vi "JSONtext Multi-step Filter.vi"() -> ()   [LabVIEW 2017] (continued)
: \"2014-12-13T11:18:37 -00:00\",\n    \"latitude\": 44.611706,\n    \"longitude\": -75.982853,\n    \"tags\": [\n      \"non\",\n      \"mollit\",\n      \"pariatur\",\n      \"ad\",\n      \"aliqua\",\n      \"do\",\n      \"laboris\"\n    ],\n    \"friends\": [\n      {\n        \"id\": 0,\n        \"name\": \"Cannon Navarro\"\n      },\n      {\n        \"id\": 1,\n        \"name\": \"Terri Byers\"\n      },\n      {\n        \"id\": 2,\n        \"name\": \"Janell Robinson\"\n      }\n    ],\n    \"greeting\": \"Hello, Carroll Kline! You have 4 unread messages.\",\n    \"favoriteFruit\": \"banana\"\n  },\n  {\n    \"_id\": \"59b53bcb034cefc38e5f718d\",\n    \"index\": 14,\n    \"guid\": \"1b75941b-966f-4520-bda0-746f5f72a03e\",\n    \"isActive\": false,\n    \"balance\": \"$2,799.30\",\n    \"picture\": \"http://placehold.it/32x32\",\n    \"age\": 32,\n    \"eyeColor\": \"brown\",\n    \"name\": \"Forbes Tran\",\n    \"gender\": \"male\",\n    \"company\": \"LYRIA\",\n    \"email\": \"forbestran@lyria.com\",\n    \"phone\": \"+1 (932) 582-3482\",\n    \"address\": \"689 Cook Street, Cleary, Iowa, 2553\",\n    \"about\": \"Occaecat tempor sint nisi amet ex veniam culpa adipisicing ad. Incididunt duis elit amet deserunt eiusmod officia occaecat eiusmod qui incididunt. Eiusmod laboris esse sit incididunt enim eu excepteur est mollit anim ad quis. Mollit nulla culpa veniam incididunt ipsum sit officia sunt aliqua reprehenderit dolor dolore. Culpa excepteur consequat magna elit id ullamco deserunt est in et irure.\\r\\n\",\n    \"registered\": \"2015-05-22T09:52:23 -01:00\",\n    \"latitude\": 9.60954,\n    \"longitude\": -42.310375,\n    \"tags\": [\n      \"mollit\",\n      \"proident\",\n      \"veniam\",\n      \"irure\",\n      \"esse\",\n      \"Lorem\",\n      \"dolore\"\n    ],\n    \"friends\": [\n      {\n        \"id\": 0,\n        \"name\": \"Leila Sims\"\n      },\n      {\n        \"id\": 1,\n        \"name\": \"Desiree Savage\"\n      },\n      {\n        \"id\": 2,\n        \"name\": \"Johnston Hensley\"\n      }\n    ],\n    \"greeting\": \"Hello, Forbes Tran! You have 3 unread messages.\",\n    \"favoriteFruit\": \"banana\"\n  },\n  {\n    \"_id\": \"59b53bcb9a6e9676f507278e\",\n    \"index\": 15,\n    \"guid\": \"3bed5db5-ef23-4804-a3e0-08b3c940d53f\",\n    \"isActive\": true,\n    \"balance\": \"$1,219.22\",\n    \"picture\": \"http://placehold.it/32x32\",\n    \"age\": 39,\n    \"eyeColor\": \"brown\",\n    \"name\": \"Carlson Klein\",\n    \"gender\": \"male\",\n    \"company\": \"AQUACINE\",\n    \"email\": \"carlsonklein@aquacine.com\",\n    \"phone\": \"+1 (978) 572-2330\",\n    \"address\": \"863 Woods Place, Movico, Wyoming, 810\",\n    \"about\": \"Do excepteur nostrud est nisi minim incididunt cillum. Et veniam do in proident deserunt minim sit. Sunt pariatur ipsum tempor elit duis sint sit non non qui laborum duis esse. Sint eiusmod irure pariatur occaecat reprehenderit anim.\\r\\n\",\n    \"registered\": \"2014-05-03T11:19:28 -01:00\",\n    \"latitude\": -56.803333,\n    \"longitude\": -128.863204,\n    \"tags\": [\n      \"tempor\",\n      \"velit\",\n      \"voluptate\",\n      \"et\",\n      \"laboris\",\n      \"consequat\",\n      \"cillum\"\n    ],\n    \"friends\": [\n      {\n        \"id\": 0,\n        \"name\": \"Liliana Sellers\"\n      },\n      {\n        \"id\": 1,\n        \"name\": \"Garcia Larsen\"\n      },\n      {\n        \"id\": 2,\n        \"name\": \"Long Fitzpatrick\"\n      }\n    ],\n    \"greeting\": \"Hello, Carlson Klein! You have 4 unread messages.\",\n    \"favoriteFruit\": \"strawberry\"\n  },\n  {\n    \"_id\": \"59b53bcbac141192de4ff36f\",\n    \"index\": 16,\n    \"guid\": \"5c96733c-76df-40fa-b2b3-d65d58dc0720\",\n    \"isActive\": true,\n    \"balance\": \"$2,144.12\",\n    \"picture\": \"http://placehold.it/32x32\",\n    \"age\": 38,\n    \"eyeColor\": \"blue\",\n    \"name\": \"Maryann Adams\",\n    \"gender\": \"female\",\n    \"company\": \"GEEKY\",\n    \"email\": \"maryannadams@geeky.com\",\n    \"phone\": \"+1 (814) 507-3036\",\n    \"address\": \"701 Albemarle Terrace, Datil, Marshall Islands, 1322\",\n    \"about\": \"Ipsum velit nostrud minim aute velit ut esse occaecat ad voluptate qui ad. Mollit pariatur ullamco Lorem quis elit incididunt anim ullamco officia laborum. Ad incididunt ut ipsum elit elit culpa magna. Nulla quis ex est elit commodo deserunt culpa culpa sint occaecat do. Consectetur irure officia culpa id ex. Et est id minim proident Lorem ea esse aute et qui. Quis enim duis minim sint elit nostrud.\\r\\n\",\n    \"registered\": \"2016-11-20T04:37:14 -00:00\",\n    \"latitude\": -61.054651,\n    \"longitude\": -110.864468,\n    \"tags\": [\n      \"excepteur\",\n      \"minim\",\n      \"amet\",\n      \"magna\",\n      \"fugiat\",\n      \"excepteur\",\n      \"consectetur\"\n    ],\n    \"friends\": [\n      {\n        \"id\": 0,\n        \"name\": \"Megan Petersen\"\n      },\n      {\n        \"id\": 1,\n        \"name\": \"Arline Solis\"\n      },\n      {\n        \"id\": 2,\n        \"name\": \"Carpenter Bishop\"\n      }\n    ],\n    \"greeting\": \"Hello, Maryann Adams! You have 4 unread messages.\",\n    \"favoriteFruit\": \"apple\"\n  },\n  {\n    \"_id\": \"59b53bcbd4794b54dacb02ff\",\n    \"index\": 17,\n    \"guid\": \"9b12691d-534a-49ef-9453-e6db5e086fa3\",\n    \"isActive\": true,\n    \"balance\": \"$1,444.83\",\n    \"picture\": \"http://placehold.it/32x32\",\n    \"age\": 23,\n    \"eyeColor\": \"brown\",\n    \"name\": \"Zelma Hooper\",\n    \"gender\": \"female\",\n    \"company\": \"ENDICIL\",\n    \"email\": \"zelmahooper@endicil.com\",\n    \"phone\": \"+1 (953) 529-2225\",\n    \"address\": \"327 Cherry Street, Sylvanite, Nevada, 1609\",\n    \"about\": \"Aliquip consectetur dolor magna irure voluptate ea. Labore id aute incididunt eiusmod ad cillum est exercitation excepteur officia cupidatat aute. Sit et magna duis duis excepteur ad est sit sint adipisicing commodo. Sint est quis amet ullamco cupidatat nisi enim sint do et.\\r\\n\",\n    \"registered\": \"2015-10-10T05:49:22 -01:00\",\n    \"latitude\": -69.361083,\n    \"longitude\": -9.671064,\n    \"tags\": [\n      \"veniam\",\n      \"officia\",\n      \"dolore\",\n      \"dolore\",\n      \"occaecat\",\n      \"excepteur\",\n      \"dolore\"\n    ],\n    \"friends\": [\n      {\n        \"id\": 0,\n        \"name\": \"Hughes Mcgowan\"\n      },\n      {\n        \"id\": 1,\n        \"name\": \"Corrine Velazquez\"\n      },\n      {\n        \"id\": 2,\n        \"name\": \"Wade Kirkland\"\n      }\n    ],\n    \"greeting\": \"Hello, Zelma Hooper! You have 6 unread messages.\",\n    \"favoriteFruit\": \"strawberry\"\n  },\n  {\n    \"_id\": \"59b53bcb68e219d872f06a49\",\n    \"index\": 18,\n    \"guid\": \"861c801f-0f15-4390-8104-311e6d6f83d8\",\n    \"isActive\": true,\n    \"balance\": \"$2,222.35\",\n    \"picture\": \"http://placehold.it/32x32\",\n    \"age\": 34,\n    \"eyeColor\": \"green\",\n    \"name\": \"Gwen Cook\",\n    \"gender\": \"female\",\n    \"company\": \"BESTO\",\n    \"email\": \"gwencook@besto.com\",\n    \"phone\": \"+1 (999) 515-3826\",\n    \"address\": \"151 Wythe Place, Hessville, North Carolina, 3410\",\n    \"about\": \"Fugiat aliqua nulla ea et do tempor ex sit mollit. Aliquip id dolor incididunt eu anim. Qui ex Lorem ut tempor veniam sit nostrud. Sint elit adipisicing laboris exercitation enim sint. Ipsum in anim quis magna. Ullamco deserunt voluptate reprehenderit tempor ea proident ea. Ea ad deserunt esse anim quis.\\r\\n\",\n    \"registered\": \"2016-01-02T10:58:42 -00:00\",\n    \"latitude\": 62.88102,\n    \"longitude\": -110.611076,\n    \"tags\": [\n      \"veniam\",\n      \"consectetur\",\n      \"consequat\",\n      \"fugiat\",\n      \"aliqua\",\n      \"incididunt\",\n      \"deserunt\"\n    ],\n    \"friends\": [\n      {\n        \"id\": 0,\n        \"name\": \"Powell Burris\"\n      },\n      {\n        \"id\": 1,\n        \"name\": \"Nina Burt\"\n      },\n      {\n        \"id\": 2,\n        \"name\": \"Brandi Barber\"\n      }\n    ],\n    \"greeting\": \"Hello, Gwen Cook! You have 4 unread messages.\",\n    \"favoriteFruit\": \"apple\"\n  },\n  {\n    \"_id\": \"59b53bcb7b31d5c7dd72738c\",\n    \"index\": 19,\n    \"guid\": \"a44d6ef3-72ce-47e3-be35-e26aef54e05c\",\n    \"isActive\": true,\n    \"balance\": \"$2,772.61\",\n    \"picture\": \"http://placehold.it/32x32\",\n    \"age\": 27,\n    \"eyeColor\": \"brown\",\n    \"name\": \"Ray Sheppard\",\n    \"gender\": \"male\",\n    \"company\": \"STEELFAB\",\n    \"email\": \"raysheppard@steelfab.com\",\n    \"phone\": \"+1 (833) 576-3166\",\n    \"address\": \"421 Noel Avenue, Fruitdale, New Mexico, 1023\",\n    \"about\": \"Nisi tempor ea nostrud reprehenderit labore Lorem proident adipisicing aliqua anim ad. Lorem id mollit nisi et minim nostrud proident commodo et dolore ex. Lorem anim eu eu sint exercitation sint.\\r\\n\",\n    \"registered\": \"2016-10-14T02:28:34 -01:00\",\n    \"latitude\": -21.473911,\n    \"longitude\": -178.75414,\n    \"tags\": [\n      \"deserunt\",\n      \"sint\",\n      \"culpa\",\n      \"mollit\",\n      \"minim\",\n      \"aute\",\n      \"dolor\"\n    ],\n    \"friends\": [\n      {\n        \"id\": 0,\n        \"name\": \"Joan Donaldson\"\n      },\n      {\n        \"id\": 1,\n        \"name\": \"Lilly Hansen\"\n      },\n      {\n        \"id\": 2,\n        \"name\": \"Francis Foster\"\n      }\n    ],\n    \"greeting\": \"Hello, Ray Sheppard! You have 1 unread messages.\",\n    \"favoriteFruit\": \"banana\"\n  },\n  {\n    \"_id\": \"59b53bcbfc475205683d24fb\",\n    \"index\": 20,\n    \"guid\": \"70656bad-68de-4581-9553-567f23d70256\",\n    \"isActive\": false,\n    \"balance\": \"$1,071.41\",\n    \"picture\": \"http://placehold.it/32x32\",\n    \"age\": 23,\n    \"eyeColor\": \"green\",\n    \"name\": \"Kerr Bowman\",\n    \"gender\": \"male\",\n    \"company\": \"SUPPORTAL\",\n    \"email\": \"kerrbowman@supportal.com\",\n    \"phone\": \"+1 (915) 525-3701\",\n    \"address\": \"387 Gallatin Place, Williston, Michigan, 658\",\n    \"about\": \"Sint nostrud qui deserunt sit tempor esse do sunt amet exercitation anim nulla. Eiusmod ex tempor in officia consequat dolor exercitation irure incididunt nulla nulla do. Mollit magna do et ea cupidatat elit ipsum adipisicing voluptate cupidatat eiusmod non.\\r\\n\",\n    \"registered\": \"2015-07-19T05:10:09 -01:00\",\n    \"latitude\": -61.588655,\n    \"longitude\": -69.987029,\n    \"tags\": [\n      \"laborum\",\n      \"laborum\",\n      \"consequat\",\n      \"ut\",\n      \"magna\",\n      \"voluptate\",\n      \"esse\"\n    ],\n    \"friends\": [\n      {\n        \"id\": 0,\n        \"name\": \"Beryl Wolfe\"\n      },\n      {\n        \"id\": 1,\n        \"name\": \"Viola Hamilton\"\n      },\n      {\n        \"id\": 2,\n        \"name\": \"Jannie Whitehead\"\n      }\n    ],\n    \"greeting\": \"Hello, Kerr Bowman! You have 2 unread messages.\",\n    \"favoriteFruit\": \"banana\"\n  },\n  {\n    \"_id\": \"59b53bcb8d287deabf6d0b79\",\n    \"index\": 21,\n    \"guid\": \"7c1a5e48-bb0e-4c13-81d4-88d15f5cbdd2\",\n    \"isActive\": false,\n    \"balance\": \"$3,025.85\",\n    \"picture\": \"http://placehold.it/32x32\",\n    \"age\": 31,\n    \"eyeColor\": \"green\",\n    \"name\": \"Aline Fleming\",\n    \"gender\": \"female\",\n    \"company\": \"COMCUR\",\n    \"email\": \"alinefleming@comcur.com\",\n    \"phone\": \"+1 (973) 454-2935\",\n    \"address\": \"736 Harbor Court, Allison, Oregon, 7524\",\n    \"about\": \"Do dolore deserunt dolor anim ex cillum ea amet ipsum in irure. Labore nisi culpa deserunt ipsum quis exercitation fugiat esse velit dolor reprehenderit. Ea id non quis ipsum officia. Enim veniam minim excepteur do dolore commodo nulla culpa irure.\\r\\n\",\n    \"registered\": \"2015-03-20T09:17:16 -00:00\",\n    \"latitude\": -85.661732,\n    \"longitude\": -109.540686,\n    \"tags\": [\n      \"laborum\",\n      \"aute\",\n      \"do\",\n      \"magna\",\n      \"do\",\n      \"Lorem\",\n      \"officia\"\n    ],\n    \"friends\": [\n      {\n        \"id\": 0,\n        \"name\": \"Corinne Rush\"\n      },\n      {\n        \"id\": 1,\n        \"name\": \"Pearlie Fuentes\"\n      },\n      {\n        \"id\": 2,\n        \"name\": \"Shelton Mendoza\"\n      }\n    ],\n    \"greeting\": \"Hello, Aline Fleming! You have 9 unread messages.\",\n    \"favoriteFruit\": \"banana\"\n  },\n  {\n    \"_id\": \"59b53bcb21bc1b9e689f86cd\",\n    \"index\": 22,\n    \"guid\": \"89e79c28-d1d3-4cf0-a7db-e52663288896\",\n    \"isActive\": false,\n    \"balance\": \"$1,913.46\",\n    \"picture\": \"http://placehold.it/32x32\",\n    \"age\": 20,\n    \"eyeColor\": \"green\",\n    \"name\": \"Stacey Hickman\",\n    \"gender\": \"female\",\n    \"company\": \"OLYMPIX\",\n    \"email\": \"staceyhickman@olympix.com\",\n    \"phone\": \"+1 (885) 484-3824\",\n    \"address\": \"738 Oxford Walk, Bagtown, Florida, 6859\",\n    \"about\": \"Occaecat in in do commodo esse aute. Consectetur voluptate amet dolore ad amet reprehenderit. Ut ullamco velit labore exercitation commodo adipisicing ea ea. Cupidatat do pariatur excepteur commodo tempor aute sint exercitation.\\r\\n\",\n    \"registered\": \"2017-06-13T05:36:22 -01:00\",\n    \"latitude\": 48.262654,\n    \"longitude\": -98.857032,\n    \"tags\": [\n      \"culpa\",\n      \"excepteur\",\n      \"irure\",\n      \"officia\",\n      \"minim\",\n      \"mollit\",\n      \"officia\"\n    ],\n    \"friends\": [\n      {\n        \"id\": 0,\n        \"name\": \"Natasha Anderson\"\n      },\n      {\n        \"id\": 1,\n        \"name\": \"Blackwell Blanchard\"\n      },\n      {\n        \"id\": 2,\n        \"name\": \"Iva Riggs\"\n      }\n    ],\n    \"greeting\": \"Hello, Stacey Hickman! You have 1 unread messages.\",\n    \"favoriteFruit\": \"banana\"\n  },\n  {\n    \"_id\": \"59b53bcbf9cf2b4cfa69d511\",\n    \"index\": 23,\n    \"guid\": \"54e3fdd1-4f8d-42dc-9828-ba8270d810c4\",\n    \"isActive\": true,\n    \"balance\": \"$1,863.08\",\n    \"picture\": \"http://placehold.it/32x32\",\n    \"age\": 30,\n    \"eyeColor\": \"brown\",\n    \"name\": \"Dora Larson\",\n    \"gender\": \"female\",\n    \"company\": \"XTH\",\n    \"email\": \"doralarson@xth.com\",\n    \"phone\": \"+1 (817) 432-2284\",\n    \"address\": \"433 Love Lane, Cliff, Minnesota, 8201\",\n    \"about\": \"Ad id pariatur nulla Lorem consequat. In veniam dolore do nisi incididunt. Mollit occaecat quis irure ut consectetur in duis culpa adipisicing in sunt consequat adipisicing.\\r\\n\",\n    \"registered\": \"2015-03-08T09:12:31 -00:00\",\n    \"latitude\": 42.824631,\n    \"longitude\": -141.172328,\n    \"tags\": [\n      \"laborum\",\n      \"ut\",\n      \"fugiat\",\n      \"veniam\",\n      \"cupidatat\",\n      \"sit\",\n      \"et\"\n    ],\n    \"friends\": [\n      {\n        \"id\": 0,\n        \"name\": \"Coffey Munoz\"\n      },\n      {\n        \"id\": 1,\n        \"name\": \"Hope Case\"\n      },\n      {\n        \"id\": 2,\n        \"name\": \"Marquez Hutchinson\"\n      }\n    ],\n    \"greeting\": \"Hello, Dora Larson! You have 9 unread messages.\",\n    \"favoriteFruit\": \"banana\"\n  },\n  {\n    \"_id\": \"59b53bcb7452ac2216503911\",\n    \"index\": 24,\n    \"guid\": \"305c5641-1f82-4362-953f-80e8de19eacf\",\n    \"isActive\": false,\n    \"balance\": \"$3,504.96\",\n    \"picture\": \"http://placehold.it/32x32\",\n    \"age\": 32,\n    \"eyeColor\": \"brown\",\n    \"name\": \"Estes Wilkins\",\n    \"gender\": \"male\",\n    \"company\": \"GUSHKOOL\",\n    \"email\": \"esteswilkins@gushkool.com\",\n    \"phone\": \"+1 (957) 533-3834\",\n    \"address\": \"168 Krier Place, Cartwright, Hawaii, 187\",\n    \"about\": \"Elit consectetur minim quis esse proident cillum cupidatat. Occaecat aute velit do Lorem ullamco esse. Duis eu sint dolore ut mollit cupidatat consectetur minim et in nostrud. Adipisicing labore incididunt id eiusmod elit reprehenderit. Ea ullamco aliquip cillum proident mollit aliqua nostrud. Dolore aliqua mollit deserunt aliqua deserunt veniam.\\r\\n\",\n    \"registered\": \"2015-06-16T05:18:07 -01:00\",\n    \"latitude\": -48.357251,\n    \"longitude\": 179.978918,\n    \"tags\": [\n      \"id\",\n      \"ullamco\",\n      \"exercitation\",\n      \"adipisicing\",\n      \"esse\",\n      \"eu\",\n      \"veniam\"\n    ],\n    \"friends\": [\n      {\n        \"id\": 0,\n        \"name\": \"Small Gibson\"\n      },\n      {\n        \"id\": 1,\n        \"name\": \"Gonzalez Potts\"\n      },\n      {\n        \"id\": 2,\n        \"name\": \"Alvarez Mcguire\"\n      }\n    ],\n    \"greeting\": \"Hello, Estes Wilkins! You have 10 unread messages.\",\n    \"favoriteFruit\": \"strawberry\"\n  },\n  {\n    \"_id\": \"59b53bcb9a5eee5c2af3c441\",\n    \"index\": 25,\n    \"guid\": \"c524b090-0f2c-4b34-b60b-c57e786f3800\",\n    \"isActive\": false,\n    \"balance\": \"$3,668.62\",\n    \"picture\": \"http://placehold.it/32x32\",\n    \"age\": 25,\n    \"eyeColor\": \"blue\",\n    \"name\": \"Betsy Leblanc\",\n    \"gender\": \"female\",\n    \"company\": \"FANFARE\",\n    \"email\": \"betsyleblanc@fanfare.com\",\n    \"phone\": \"+1 (879) 416-2965\",\n    \"address\": \"393 Prospect Avenue, Thermal, Pennsylvania, 1021\",\n    \"about\": \"Voluptate do duis amet ut dolor eiusmod nisi deserunt fugiat consequat. Proident officia reprehenderit voluptate nisi qui anim incididunt reprehenderit id. Culpa dolor adipisicing eu duis aute occaecat irure adipisicing aliqua. Duis sunt eiusmod occaecat ipsum do anim elit consectetur magna irure elit. Laboris nisi ea in elit sit pariatur est nostrud amet.\\r\\n\",\n    \"registered\": \"2014-08-22T09:02:28 -01:00\",\n    \"latitude\": -20.158386,\n    \"longitude\": 36.762045,\n    \"tags\": [\n      \"veniam\",\n      \"id\",\n      \"deserunt\",\n      \"aliquip\",\n      \"labore\",\n      \"consectetur\",\n      \"voluptate\"\n    ],\n    \"friends\": [\n      {\n        \"id\": 0,\n        \"name\": \"Esperanza Meadows\"\n      },\n      {\n        \"id\": 1,\n        \"name\": \"Jacquelyn Booker\"\n      },\n      {\n        \"id\": 2,\n        \"name\": \"Justine Higgins\"\n      }\n    ],\n    \"greeting\": \"Hello, Betsy Leblanc! You have 4 unread messages.\",\n    \"favoriteFruit\": \"apple\"\n  },\n  {\n    \"_id\": \"59b53bcb8b6a556b334bc9b5\",\n    \"index\": 26,\n    \"guid\": \"c4d258cd-4b15-4f62-a48a-45ae318736cc\",\n    \"isActive\": false,\n    \"balance\": \"$1,381.58\",\n    \"picture\": \"http://placehold.it/32x32\",\n    \"age\": 27,\n    \"eyeColor\": \"brown\",\n    \"name\": \"Gabriela Knowles\",\n    \"gender\": \"female\",\n    \"company\": \"GOLISTIC\",\n    \"email\": \"gabrielaknowles@golistic.com\",\n    \"phone\": \"+1 (984) 554-3557\",\n    \"address\": \"108 Gerry Street, Ryderwood, Virginia, 954\",\n    \"about\": \"Nostrud adipisicing duis cupidatat mollit incididunt velit commodo ea elit commodo. Magna duis consectetur labore ullamco ullamco. Proident enim ad enim ex aliquip dolor duis non ipsum nulla do enim nostrud cillum. Anim cillum labore mollit proident cillum esse culpa consequat id exercitation dolor officia sunt. Anim ipsum deserunt enim proident cupidatat tempor.\\r\\n\",\n    \"registered\": \"2017-03-10T12:46:33 -00:00\",\n    \"latitude\": -72.605964,\n    \"longitude\": -124.787196,\n    \"tags\": [\n      \"in\",\n      \"dolore\",\n      \"elit\",\n      \"magna\",\n      \"in\",\n      \"occaecat\",\n      \"ipsum\"\n    ],\n    \"friends\": [\n      {\n        \"id\": 0,\n        \"name\": \"Shannon Nolan\"\n      },\n      {\n        \"id\": 1,\n        \"name\": \"Leann Herrera\"\n      },\n      {\n        \"id\": 2,\n        \"name\": \"Sheppard Frost\"\n      }\n    ],\n    \"greeting\": \"Hello, Gabriela Knowles! You have 6 unread messages.\",\n    \"favoriteFruit\": \"banana\"\n  },\n  {\n    \"_id\": \"59b53bcb93de39cd0c0af940\",\n    \"index\": 27,\n    \"guid\": \"0f0552d9-e7b3-4c57-b6c7-1e2135a1104f\",\n    \"isActive\": false,\n    \"balance\": \"$3,811.17\",\n    \"picture\": \"http://placehold.it/32x32\",\n    \"age\": 38,\n    \"eyeColor\": \"brown\",\n    \"name\": \"Merrill Ray\",\n    \"gender\": \"male\",\n    \"company\": \"SOLAREN\",\n    \"email\": \"merrillray@solaren.com\",\n    \"phone\": \"+1 (835) 524-2354\",\n    \"address\": \"227 Seacoast Terrace, Waterford, Kansas, 9740\",\n    \"about\": \"Magna eiusmod duis pariatur eiusmod minim et officia sit amet ipsum ut sint magna Lorem. Nisi velit sit adipisicing deserunt voluptate consectetur dolor officia voluptate elit adipisicing sit. Sint dolore occaecat ea duis voluptate duis sint ullamco in quis pariatur irure. Ipsum magna voluptate nulla deserunt eiusmod consectetur ut tempor qui pariatur quis duis. Lorem dolore qui adipisicing pariatur mollit cillum sunt nisi id deserunt tempor nisi amet. Sit cillum nisi dolore magna exercitation anim ad id consequat duis.\\r\\n\",\n    \"registered\": \"2016-06-15T02:30:18 -01:00\",\n    \"latitude\": 82.245484,\n    \"longitude\": -22.28782,\n    \"tags\": [\n      \"quis\",\n      \"pariatur\",\n      \"nisi\",\n      \"culpa\",\n      \"ut\",\n      \"minim\",\n      \"amet\"\n    ],\n    \"friends\": [\n      {\n        \"id\": 0,\n        \"name\": \"Fleming Rosario\"\n      },\n      {\n        \"id\": 1,\n        \"name\": \"Mcconnell Griffin\"\n      },\n      {\n        \"id\": 2,\n        \"name\": \"Marian Bradley\"\n      }\n    ],\n    \"greeting\": \"Hello, Merrill Ray! You have 3 unread messages.\",\n    \"favoriteFruit\": \"strawberry\"\n  },\n  {\n    \"_id\": \"59b53bcb56ebb2118edadabb\",\n    \"index\": 28,\n    \"guid\": \"31fd77e0-df37-4030-b598-6469f87deaaa\",\n    \"isActive\": false,\n    \"balance\": \"$1,128.38\",\n    \"picture\": \"http://placehold.it/32x32\",\n    \"age\": 22,\n    \"eyeColor\": \"green\",\n    \"name\": \"Cunningham Blevins\",\n    \"gender\": \"male\",\n    \"company\": \"SHOPABOUT\",\n    \"email\": \"cunninghamblevins@shopabout.com\",\n    \"phone\": \"+1 (960) 458-2822\",\n    \"address\": \"730 Llama Court, Riner, Puerto Rico, 7836\",\n    \"about\": \"Dolor quis officia nulla dolor amet sint excepteur enim esse est do. Eu ex ut aliquip velit do sint ullamco laborum. Occaecat eiusmod eiusmod velit adipisicing sit. Mollit eu pariatur eu consequat dolore irure fugiat sunt eiusmod cillum duis adipisicing eiusmod. Do commodo nisi irure cillum magna nulla enim aliqua dolor ullamco dolore pariatur.\\r\\n\",\n    \"registered\": \"2016-09-06T04:22:46 -01:00\",\n    \"latitude\": 83.759644,\n    \"longitude\": -43.131498,\n    \"tags\": [\n      \"velit\",\n      \"fugiat\",\n      \"dolor\",\n      \"ad\",\n      \"elit\",\n      \"dolore\",\n      \"ea\"\n    ],\n    \"friends\": [\n      {\n        \"id\": 0,\n        \"name\": \"Sanford Shannon\"\n      },\n      {\n        \"id\": 1,\n        \"name\": \"Burt Cherry\"\n      },\n      {\n        \"id\": 2,\n        \"name\": \"Kline Hale\"\n      }\n    ],\n    \"greeting\": \"Hello, Cunningham Blevins! You have 10 unread messages.\",\n    \"favoriteFruit\": \"strawberry\"\n  },\n  {\n    \"_id\": \"59b53bcb90a0cd7d08d9bf70\",\n    \"index\": 29,\n    \"guid\": \"8fb07447-f204-4b08-975d-44052bc193eb\",\n    \"isActive\": false,\n    \"balance\": \"$3,739.37\",\n    \"picture\": \"http://placehold.it/32x32\",\n    \"age\": 36,\n    \"eyeColor\": \"brown\",\n    \"name\": \"Bonner Lane\",\n    \"gender\": \"male\",\n    \"company\": \"COMVEY\",\n    \"email\": \"bonnerlane@comvey.com\",\n    \"phone\": \"+1 (847) 514-2794\",\n    \"address\": \"269 Dupont Street, Cedarville, South Carolina, 6587\",\n    \"about\": \"Velit Lorem magna deserunt minim ea exercitation quis veniam. Culpa cillum do aliquip exercitation enim aute in incididunt nostrud esse nostrud ullamco in. Amet mollit laborum eu laborum magna. Duis ad proident cillum esse fugiat enim est sit commodo. Dolore consectetur ut duis deserunt elit aliqua ad fugiat consectetur. Est aute aliquip ea consequat reprehenderit eiusmod. Consectetur tempor consequat duis voluptate mollit elit labore voluptate do cillum ex.\\r\\n\",\n    \"registered\": \"2017-02-20T02:31:32 -00:00\",\n    \"latitude\": -71.168208,\n    \"longitude\": -127.709761,\n    \"tags\": [\n      \"voluptate\",\n      \"consequat\",\n      \"incididunt\",\n      \"occaecat\",\n      \"amet\",\n      \"consequat\",\n      \"id\"\n    ],\n    \"friends\": [\n      {\n        \"id\": 0,\n        \"name\": \"Josie Horne\"\n      },\n      {\n        \"id\": 1,\n        \"name\": \"Nichole Weiss\"\n      },\n      {\n        \"id\": 2,\n        \"name\": \"Kristina Davidson\"\n      }\n    ],\n    \"greeting\": \"Hello, Bonner Lane! You have 3 unread messages.\",\n    \"favoriteFruit\": \"apple\"\n  },\n  {\n    \"_id\": \"59b53bcb35a25f2270b16071\",\n    \"index\": 30,\n    \"guid\": \"267938cb-8119-471f-85af-aa7a668d65fd\",\n    \"isActive\": false,\n    \"balance\": \"$2,354.36\",\n    \"picture\": \"http://placehold.it/32x32\",\n    \"age\": 35,\n    \"eyeColor\": \"blue\",\n    \"name\": \"Nielsen Burnett\",\n    \"gender\": \"male\",\n    \"company\": \"TURNABOUT\",\n    \"email\": \"nielsenburnett@turnabout.com\",\n    \"phone\": \"+1 (901) 404-2369\",\n    \"address\": \"499 Hart Place, Chesterfield, Mississippi, 6896\",\n    \"about\": \"Sunt magna sint ea deserunt reprehenderit aliqua in et proident. Minim consectetur dolore et commodo. Voluptate consectetur qui occaecat dolore eiusmod proident fugiat aute nulla id ad culpa exercitation occaecat.\\r\\n\",\n    \"registered\": \"2015-02-20T12:03:11 -00:00\",\n    \"latitude\": -46.775808,\n    \"longitude\": 173.193033,\n    \"tags\": [\n      \"enim\",\n      \"dolor\",\n      \"duis\",\n      \"Lorem\",\n      \"in\",\n      \"reprehenderit\",\n      \"ullamco\"\n    ],\n    \"friends\": [\n      {\n        \"id\": 0,\n        \"name\": \"Barlow Mcfadden\"\n      },\n      {\n        \"id\": 1,\n        \"name\": \"Clarissa Charles\"\n      },\n      {\n        \"id\": 2,\n        \"name\": \"Bray Patel\"\n      }\n    ],\n    \"greeting\": \"Hello, Nielsen Burnett! You have 7 unread messages.\",\n    \"favoriteFruit\": \"strawberry\"\n  },\n  {\n    \"_id\": \"59b53bcbe85d478fcadd3603\",\n    \"index\": 31,\n    \"guid\": \"3be04d8f-e807-4ad6-8ebd-c23cdbfe3dc4\",\n    \"isActive\": false,\n    \"balance\": \"$1,972.40\",\n    \"picture\": \"http://placehold.it/32x32\",\n    \"age\": 37,\n    \"eyeColor\": \"blue\",\n    \"name\": \"Elaine Allison\",\n    \"gender\": \"female\",\n    \"company\": \"QUANTASIS\",\n    \"email\": \"elaineallison@quantasis.com\",\n    \"phone\": \"+1 (981) 596-2824\",\n    \"address\": \"921 Kent Avenue, Breinigsville, Wisconsin, 3750\",\n    \"about\": \"Minim cillum ea irure officia. Irure in dolor ea veniam adipisicing sint nisi amet ipsum excepteur nisi excepteur est deserunt. Consequat voluptate mollit sint magna Lorem in nulla proident Lorem. Proident est id esse ad ea. Dolore Lorem aliquip officia veniam anim velit et id ullamco et dolor eu aliqua quis. Dolore magna est mollit in ut ea voluptate nostrud do aliquip. In reprehenderit non eiusmod veniam ex.\\r\\n\",\n    \"registered\": \"2017-03-24T04:15:39 -00:00\",\n    \"latitude\": 7.656665,\n    \"longitude\": 56.755826,\n    \"tags\": [\n      \"nisi\",\n      \"labore\",\n      \"fugiat\",\n      \"ex\",\n      \"reprehenderit\",\n      \"nisi\",\n      \"sint\"\n    ],\n    \"friends\": [\n      {\n        \"id\": 0,\n        \"name\": \"Alta Bruce\"\n      },\n      {\n        \"id\": 1,\n        \"name\": \"Cora Ruiz\"\n      },\n      {\n        \"id\": 2,\n        \"name\": \"Mercer Barron\"\n      }\n    ],\n    \"greeting\": \"Hello, Elaine Allison! You have 1 unread messages.\",\n    \"favoriteFruit\": \"banana\"\n  },\n  {\n    \"_id\": \"59b53bcbf5dcc9341b3c298d\",\n    \"index\": 32,\n    \"guid\": \"bf62375b-123f-4c02-85e3-3a78c18e6f70\",\n    \"isActive\": false,\n    \"balance\": \"$1,895.96\",\n    \"picture\": \"http://placehold.it/32x32\",\n    \"age\": 28,\n    \"eyeColor\": \"brown\",\n    \"name\": \"Christa Robertson\",\n    \"gender\": \"female\",\n    \"company\": \"ICOLOGY\",\n    \"email\": \"christarobertson@icology.com\",\n    \"phone\": \"+1 (888) 410-3337\",\n    \"address\": \"989 Clara Street, Ogema, Indiana, 2922\",\n    \"about\": \"Enim mollit officia occaecat non nostrud ad cupidatat amet. Sunt ipsum proident consectetur voluptate id excepteur id magna. Do commodo culpa id esse officia cupidatat dolore duis non laboris veniam. Laboris ad dolor qui anim et ut dolor excepteur irure elit adipisicing ex labore eiusmod. Sunt minim velit nostrud irure quis consequat officia fugiat amet ipsum. Nostrud laboris do fugiat proident reprehenderit duis exercitation aute enim ex ullamco proident. Qui sint adipisicing occaecat aliqua non culpa esse id dolor voluptate ipsum deserunt in.\\r\\n\",\n    \"registered\": \"2015-02-16T07:12:55 -00:00\",\n    \"latitude\": 52.102423,\n    \"longitude\": -24.794434,\n    \"tags\": [\n      \"dolore\",\n      \"fugiat\",\n      \"aliqua\",\n      \"minim\",\n      \"pariatur\",\n      \"laborum\",\n      \"qui\"\n    ],\n    \"friends\": [\n      {\n        \"id\": 0,\n        \"name\": \"Cathy Cohen\"\n      },\n      {\n        \"id\": 1,\n        \"name\": \"Shawna Green\"\n      },\n      {\n        \"id\": 2,\n        \"name\": \"Ward Mckay\"\n      }\n    ],\n    \"greeting\": \"Hello, Christa Robertson! You have 9 unread messages.\",\n    \"favoriteFruit\": \"banana\"\n  },\n  {\n    \"_id\": \"59b53bcb8f369a2e50811288\",\n    \"index\": 33,\n    \"guid\": \"74275f14-281e-4519-a0c4-b708fa901d88\",\n    \"isActive\": true,\n    \"balance\": \"$2,269.82\",\n    \"picture\": \"http://placehold.it/32x32\",\n    \"age\": 36,\n    \"eyeColor\": \"green\",\n    \"name\": \"Castillo Kerr\",\n    \"gender\": \"male\",\n    \"company\": \"ZENTHALL\",\n    \"email\": \"castillokerr@zenthall.com\",\n    \"phone\": \"+1 (964) 406-2670\",\n    \"address\": \"210 Campus Road, Templeton, Tennessee, 2482\",\n    \"about\": \"Irure ut nisi adipisicing non duis mollit. Tempor deserunt ut nostrud ipsum enim dolore Lorem labore. Duis sint magna nisi et anim ex. Ea eu exercitation est laboris nostrud qui eiusmod. Ullamco amet ut Lorem eu adipisicing incididunt qui aliquip pariatur sint proident anim voluptate veniam. Excepteur aute velit deserunt deserunt et ex elit excepteur enim reprehenderit. Commodo ad aliquip Lorem excepteur reprehenderit quis in ea sint esse proident.\\r\\n\",\n    \"registered\": \"2016-05-03T04:24:26 -01:00\",\n    \"latitude\": -38.877683,\n    \"longitude\": -171.766918,\n    \"tags\": [\n      \"officia\",\n      \"aliquip\",\n      \"consequat\",\n      \"voluptate\",\n      \"cillum\",\n      \"do\",\n      \"officia\"\n    ],\n    \"friends\": [\n      {\n        \"id\": 0,\n        \"name\": \"Cara Hoffman\"\n      },\n      {\n        \"id\": 1,\n        \"name\": \"Joyner Beasley\"\n      },\n      {\n        \"id\": 2,\n        \"name\": \"Lucy Grimes\"\n      }\n    ],\n    \"greeting\": \"Hello, Castillo Kerr! You have 9 unread messages.\",\n    \"favoriteFruit\": \"strawberry\"\n  },\n  {\n    \"_id\": \"59b53bcbb2ac6162cf8d89a7\",\n    \"index\": 34,\n    \"guid\": \"3d62cd17-ac67-4b71-a5da-4ccef6cce1d0\",\n    \"isActive\": false,\n    \"balance\": \"$1,731.00\",\n    \"picture\": \"http://placehold.it/32x32\",\n    \"age\": 24,\n    \"eyeColor\": \"blue\",\n    \"name\": \"Melissa Gregory\",\n    \"gender\": \"female\",\n    \"company\": \"UPLINX\",\n    \"email\": \"melissagregory@uplinx.com\",\n    \"phone\": \"+1 (907) 532-2994\",\n    \"address\": \"394 Miller Avenue, Cashtown, Georgia, 520\",\n    \"about\": \"Consequat mollit occaecat proident officia reprehenderit. Ipsum minim ex reprehenderit et reprehenderit sunt. Esse ea quis nulla do. Cupidatat sit et tempor tempor voluptate qui est ad. Ad magna adipisicing excepteur excepteur ad quis. Fugiat laborum adipisicing do commodo ex qui ut minim ipsum commodo irure ex ea. Fugiat ad anim dolor do adipisicing veniam laboris laboris nostrud reprehenderit mollit eiusmod dolore laboris.\\r\\n\",\n    \"registered\": \"2016-03-22T12:23:21 -00:00\",\n    \"latitude\": -13.24058,\n    \"longitude\": 174.343852,\n    \"tags\": [\n      \"aliqua\",\n      \"veniam\",\n      \"do\",\n      \"tempor\",\n      \"voluptate\",\n      \"officia\",\n      \"id\"\n    ],\n    \"friends\": [\n      {\n        \"id\": 0,\n        \"name\": \"Mccall Baker\"\n      },\n      {\n        \"id\": 1,\n        \"name\": \"Elena Raymond\"\n      },\n      {\n        \"id\": 2,\n        \"name\": \"Harvey Hubbard\"\n      }\n    ],\n    \"greeting\": \"Hello, Melissa Gregory! You have 7 unread messages.\",\n    \"favoriteFruit\": \"banana\"\n  },\n  {\n    \"_id\": \"59b53bcb9bea1476ae4824c8\",\n    \"index\": 35,\n    \"guid\": \"705c7090-a759-43dc-b18c-63ad736d29ca\",\n    \"isActive\": false,\n    \"balance\": \"$2,004.78\",\n    \"picture\": \"http://placehold.it/32x32\",\n    \"age\": 37,\n    \"eyeColor\": \"brown\",\n    \"name\": \"Lancaster Welch\",\n    \"gender\": \"male\",\n    \"company\": \"JIMBIES\",\n    \"email\": \"lancasterwelch@jimbies.com\",\n    \"phone\": \"+1 (961) 509-2893\",\n    \"address\": \"477 Crystal Street, Lindcove, New Hampshire, 655\",\n    \"about\": \"Anim ex duis laboris non ullamco non deserunt magna ex voluptate mollit in excepteur. Sit excepteur proident ad magna esse elit veniam qui ad veniam cupidatat non duis. Eiusmod laboris id cupidatat exercitation quis adipisicing sunt eiusmod enim magna. Qui aliqua qui dolore enim veniam consequat ea cillum cupidatat voluptate excepteur in. Eu culpa anim veniam nisi officia consectetur ut exercitation fugiat quis sit ipsum enim quis. Lorem ut magna in sit.\\r\\n\",\n    \"registered\": \"2016-07-01T05:06:00 -01:00\",\n    \"latitude\": 29.49636,\n    \"longitude\": -45.617538,\n    \"tags\": [\n      \"adipisicing\",\n      \"enim\",\n      \"do\",\n      \"culpa\",\n      \"esse\",\n      \"proident\",\n      \"velit\"\n    ],\n    \"friends\": [\n      {\n        \"id\": 0,\n        \"name\": \"Whitehead Moss\"\n      },\n      {\n        \"id\": 1,\n        \"name\": \"Melisa Bridges\"\n      },\n      {\n        \"id\": 2,\n        \"name\": \"Helene Barrett\"\n      }\n    ],\n    \"greeting\": \"Hello, Lancaster Welch! You have 4 unread messages.\",\n    \"favoriteFruit\": \"strawberry\"\n  },\n  {\n    \"_id\": \"59b53bcb1dfb6733db2fc827\",\n    \"index\": 36,\n    \"guid\": \"0d80f8b7-650a-4492-b9ae-8c5d36bf2d83\",\n    \"isActive\": true,\n    \"balance\": \"$3,087.53\",\n    \"picture\": \"http://placehold.it/32x32\",\n    \"age\": 21,\n    \"eyeColor\": \"brown\",\n    \"name\": \"Clemons Juarez\",\n    \"gender\": \"male\",\n    \"company\": \"EMERGENT\",\n    \"email\": \"clemonsjuarez@emergent.com\",\n    \"phone\": \"+1 (899) 574-2444\",\n    \"address\": \"962 Seagate Avenue, Diaperville, Louisiana, 9282\",\n    \"about\": \"Labore adipisicing in enim eu laboris veniam minim sit do velit. Nulla amet ullamco anim cupidatat. Aliquip officia laborum nulla nisi aliqua dolore elit aute tempor ut culpa commodo. Esse cupidatat officia pariatur pariatur.\\r\\n\",\n    \"registered\": \"2015-07-29T04:09:12 -01:00\",\n    \"latitude\": 16.025236,\n    \"longitude\": -68.678922,\n    \"tags\": [\n      \"et\",\n      \"sunt\",\n      \"enim\",\n      \"dolor\",\n      \"labore\",\n      \"nostrud\",\n      \"adipisicing\"\n    ],\n    \"friends\": [\n      {\n        \"id\": 0,\n        \"name\": \"Dorothea Barnett\"\n      },\n      {\n        \"id\": 1,\n        \"name\": \"Terrie Knox\"\n      },\n      {\n        \"id\": 2,\n        \"name\": \"Dodson Dale\"\n      }\n    ],\n    \"greeting\": \"Hello, Clemons Juarez! You have 7 unread messages.\",\n    \"favoriteFruit\": \"apple\"\n  },\n  {\n    \"_id\": \"59b53bcba7232f419ad64f14\",\n    \"index\": 37,\n    \"guid\": \"15bec63f-2a77-45db-a3cf-11092f20cb9e\",\n    \"isActive\": false,\n    \"balance\": \"$3,716.74\",\n    \"picture\": \"http://placehold.it/32x32\",\n    \"age\": 29,\n    \"eyeColor\": \"green\",\n    \"name\": \"Hillary Waller\",\n    \"gender\": \"female\",\n    \"company\": \"MUSIX\",\n    \"email\": \"hillarywaller@musix.com\",\n    \"phone\": \"+1 (947) 549-3976\",\n    \"address\": \"601 Kay Court, Rockhill, Oklahoma, 5198\",\n    \"about\": \"Sit reprehenderit ad mollit reprehenderit do aliquip fugiat aute consectetur eu excepteur eiusmod dolor Lorem. Deserunt consectetur ex et deserunt velit quis excepteur labore deserunt cillum. Dolore mollit qui proident minim eiusmod.\\r\\n\",\n    \"registered\": \"2015-10-22T03:23:57 -01:00\",\n    \"latitude\": 2.128634,\n    \"longitude\": 43.198503,\n    \"tags\": [\n      \"duis\",\n      \"non\",\n      \"dolore\",\n      \"aliqua\",\n      \"culpa\",\n      \"proident\",\n      \"sint\"\n    ],\n    \"friends\": [\n      {\n        \"id\": 0,\n        \"name\": \"Vega Lawson\"\n      },\n      {\n        \"id\": 1,\n        \"name\": \"Phelps Wolf\"\n      },\n      {\n        \"id\": 2,\n        \"name\": \"Gloria Mcmillan\"\n      }\n    ],\n    \"greeting\": \"Hello, Hillary Waller! You have 10 unread messages.\",\n    \"favoriteFruit\": \"apple\"\n  },\n  {\n    \"_id\": \"59b53bcb1344ea6331b52625\",\n    \"index\": 38,\n    \"guid\": \"561edd27-6d57-4a6f-956c-f3bf54efe435\",\n    \"isActive\": true,\n    \"balance\": \"$3,213.23\",\n    \"picture\": \"http://placehold.it/32x32\",\n    \"age\": 32,\n    \"eyeColor\": \"brown\",\n    \"name\": \"Jackie Lott\",\n    \"gender\": \"female\",\n    \"company\": \"ORBIN\",\n    \"email\": \"jackielott@orbin.com\",\n    \"phone\": \"+1 (825) 509-2344\",\n    \"address\": \"921 Frost Street, Dubois, Alaska, 1796\",\n    \"about\": \"Reprehenderit veniam Lorem ea do proident in fugiat aliqua. Id proident nostrud aliqua tempor reprehenderit eiusmod ullamco velit duis. Anim ipsum nulla reprehenderit do exercitation consequat nisi in commodo qui fugiat nostrud.\\r\\n\",\n    \"registered\": \"2017-08-19T04:32:54 -01:00\",\n    \"latitude\": 23.292166,\n    \"longitude\": 35.845555,\n    \"tags\": [\n      \"dolore\",\n      \"veniam\",\n      \"labore\",\n      \"et\",\n      \"culpa\",\n      \"est\",\n      \"officia\"\n    ],\n    \"friends\": [\n      {\n        \"id\": 0,\n        \"name\": \"Diaz Warren\"\n      },\n      {\n        \"id\": 1,\n        \"name\": \"Sullivan Watkins\"\n      },\n      {\n        \"id\": 2,\n        \"name\": \"Maynard Page\"\n      }\n    ],\n    \"greeting\": \"Hello, Jackie Lott! You have 4 unread messages.\",\n    \"favoriteFruit\": \"apple\"\n  },\n  {\n    \"_id\": \"59b53bcb21e1aba2d54ad2f8\",\n    \"index\": 39,\n    \"guid\": \"c9ee8206-d3bd-48ae-9fda-5b5529ac4057\",\n    \"isActive\": false,\n    \"balance\": \"$3,035.61\",\n    \"picture\": \"http://placehold.it/32x32\",\n    \"age\": 29,\n    \"eyeColor\": \"green\",\n    \"name\": \"Flynn Pruitt\",\n    \"gender\": \"male\",\n    \"company\": \"ORBEAN\",\n    \"email\": \"flynnpruitt@orbean.com\",\n    \"phone\": \"+1 (866) 596-2533\",\n    \"address\": \"274 Ridgewood Place, Durham, North Dakota, 3534\",\n    \"about\": \"Commodo sint irure deserunt Lorem laboris laborum mollit ea ipsum incididunt laboris adipisicing proident. Velit tempor minim et occaecat exercitation et commodo consequat velit. Minim irure esse ullamco commodo labore ex mollit esse. Ipsum nostrud est ex Lorem culpa.\\r\\n\",\n    \"registered\": \"2015-06-20T09:17:37 -01:00\",\n    \"latitude\": -50.018521,\n    \"longitude\": 165.121492,\n    \"tags\": [\n      \"irure\",\n      \"ea\",\n      \"quis\",\n      \"dolore\",\n      \"irure\",\n      \"aliqua\",\n      \"pariatur\"\n    ],\n    \"friends\": [\n      {\n
